vi "WriteGroupedDigitalOutputs.vi"(8 "error in (no error)":errorcluster, 10 "data":u32, 11 "DigitalOutput_Simulation In":refnum<class "TesteractHAL_DigitalOutput_Simulation.lvclass">) -> (0 "error out":errorcluster, 3 "DigitalOutput_Simulation Out":refnum<class "TesteractHAL_DigitalOutput_Simulation.lvclass">)   [LabVIEW 2017, in "TesteractHAL_DigitalOutput_Simulation.lvlib" / "TesteractHAL_DigitalOutput_Simulation.lvclass"]
doc: "Write a single digital channel where the number represents the bits to set on the digital signal."
uses:
  TesteractHAL_DigitalOutput_Simulation.lvclass
  TesteractHAL_DigitalOutput_Simulation.lvclass/TesteractHAL_DigitalOutput_Simulation.ctl
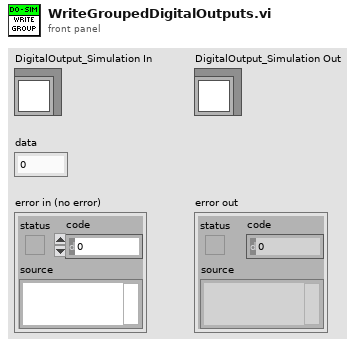
[diagram p1: front panel]
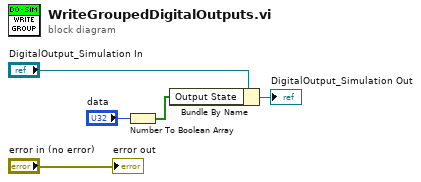
[diagram p0: block diagram]
diagram:
  n1 = Number To Boolean Array(number="data") -> (Boolean array=w1:bool[])
  n2 = Bundle By Name(cluster="DigitalOutput_Simulation In", "Output State"=w1) -> (→"DigitalOutput_Simulation Out":refnum<class "TesteractHAL_DigitalOutput_Simulation.lvclass">)
  "error out" <- "error in (no error)"
